vi "Switch Plugin Subpanel.vi"(8 "error in (no error)":errorcluster, 9 "Calling VI":refnum<vi>, 10 "Plugin Info":T1 {"Node Status"."Monitor Doubles"."4" format="%#_9g"; "Node Status"."Monitor Doubles"."3" format="%#_9g"; "Node Status"."Monitor Doubles"."2" format="%#_9g"; "Node Status"."Monitor Doubles"."1" format="%#_9g"; "Node Status"."Timing Statistics (us)"."Period"."Avg" format="%_6g"}, 11 "CIF_UI in":refnum<class "CIF_Manager_UI.lvclass">) -> (0 "error out":errorcluster, 1 "Remove Subpanel":bool, 2 "VI Reference":refnum<vi>, 3 "CIF_UI out":refnum<class "CIF_Manager_UI.lvclass">)   [LabVIEW 2021, in "CIF_Manager_UI.lvclass"]
uses:
  CIF_Manager_UI.lvclass
  C:/Program Files/National Instruments/LabVIEW 2021/vi.lib/CIF Foundation/CIF Core/CIFUI/CIF_UI.lvclass
  Typedef/PluginInfo.ctl
  <vilib>/CIF Foundation/CIF Core/CIFCore/Common/Typedef/Version Simple.ctl
  <vilib>/CIF Foundation/CIF Core/CIFCore/Common/Typedef/gRPC Reported Plugin Status.ctl
  <vilib>/CIF Foundation/CIF Core/CIFCore/Common/Typedef/Plugin State.ctl
  <vilib>/CIF Foundation/CIF Core/CIFCore/Common/Typedef/Timing Statistics.ctl
  <vilib>/CIF Foundation/CIF Core/CIFCore/Common/Typedef/Timing Stats Base.ctl
  <vilib>/CIF Foundation/CIF Core/CIFCore/Common/Typedef/FIFO Statistics.ctl
  <vilib>/CIF Foundation/CIF Core/CIFCore/Common/Typedef/Simple Error.ctl
  <vilib>/CIF Foundation/CIF Core/CIFCore/Common/Typedef/Monitor Doubles.ctl
  <vilib>/CIF Foundation/CIF Core/CIFCore/Common/Typedef/Monitor U64.ctl
  <vilib>/CIF Foundation/CIF Core/CIFCore/Common/Typedef/Monitor I64.ctl
  <vilib>/CIF Foundation/CIF Core/CIFUI/CIF_UI.lvclass/CIF_UI.ctl
  <vilib>/CIF Foundation/CIF Core/CIFUI/Accessors/Read Plugin Subpanel Map.vi
  <vilib>/Utility/LVLibp/Get Exported File List.vi
  <vilib>/Utility/LVLibp/Get Exported File Path.vi
  <vilib>/Utility/LVLibp/Packed Library Path.vi
  <vilib>/CIF Foundation/CIF Core/CIFUI/CIF_UI.lvclass
  <vilib>/CIF Foundation/CIF Core/CIFCore/Common/CIFCoreCommon.lvlib
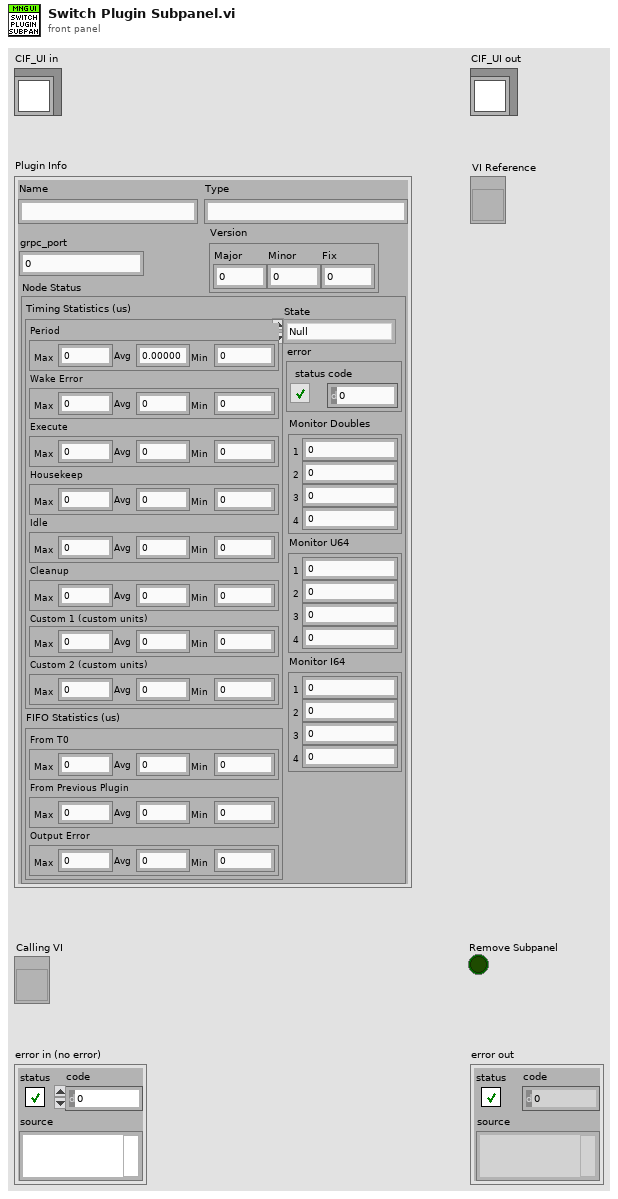
[diagram p1: front panel]
types:
  T1 = typedef "CIF_Manager_UI.lvclass/PluginInfo.ctl" = cluster{"Name":string, "Type":string, "grpc_port":i32, "Version":T2, "Node Status":T3}
  T2 = typedef "CIFCoreCommon.lvlib/Version Simple.ctl" = cluster{"Major":i32, "Minor":i32, "Fix":i32}
  T3 = typedef "CIFCoreCommon.lvlib/gRPC Reported Plugin Status.ctl" = cluster{"State":T4, "Timing Statistics (us)":T5, "FIFO Statistics (us)":T7, "error":T8, "Monitor Doubles":T9, "Monitor U64":T10, "Monitor I64":T11}
  T4 = typedef "CIFCoreCommon.lvlib/Plugin State.ctl" = enum32{"Null", "Creating", "Listening", "Running", "CleaningUp", "Destroying", "Prepared", "FTE_Run"}
  T5 = typedef "CIFCoreCommon.lvlib/Timing Statistics.ctl" = cluster{"Period":T6, "Wake Error":T6, "Execute":T6, "Housekeep":T6, "Idle":T6, "Cleanup":T6, "Custom 1 (custom units)":T6, "Custom 2 (custom units)":T6}
  T6 = typedef "CIFCoreCommon.lvlib/Timing Stats Base.ctl" = cluster{"Max":i64, "Avg":dbl, "Min":i64}
  T7 = typedef "CIFCoreCommon.lvlib/FIFO Statistics.ctl" = cluster{"From T0":T6, "From Previous Plugin":T6, "Output Error":T6}
  T8 = typedef "CIFCoreCommon.lvlib/Simple Error.ctl" = cluster{"status":bool, "code":i32}
  T9 = typedef "CIFCoreCommon.lvlib/Monitor Doubles.ctl" = cluster{"1":dbl, "2":dbl, "3":dbl, "4":dbl}
  T10 = typedef "CIFCoreCommon.lvlib/Monitor U64.ctl" = cluster{"1":u64, "2":u64, "3":u64, "4":u64}
  T11 = typedef "CIFCoreCommon.lvlib/Monitor I64.ctl" = cluster{"1":i64, "2":i64, "3":i64, "4":i64}
  T12 = typedef "CIF_UI.lvclass/Plugin Subpanel Map.ctl" = map{i32, T13}
  T13 = typedef "CIF_UI.lvclass/Subpanel Data.ctl" = cluster{"VI Reference":refnum<vi>, "Plugin Subpanel Events":T14}
  T14 = typedef "CIF_UI.lvclass/Plugin Subpanel Events.ctl" = cluster{"Plugin Shutdown":refnum<user-event>}
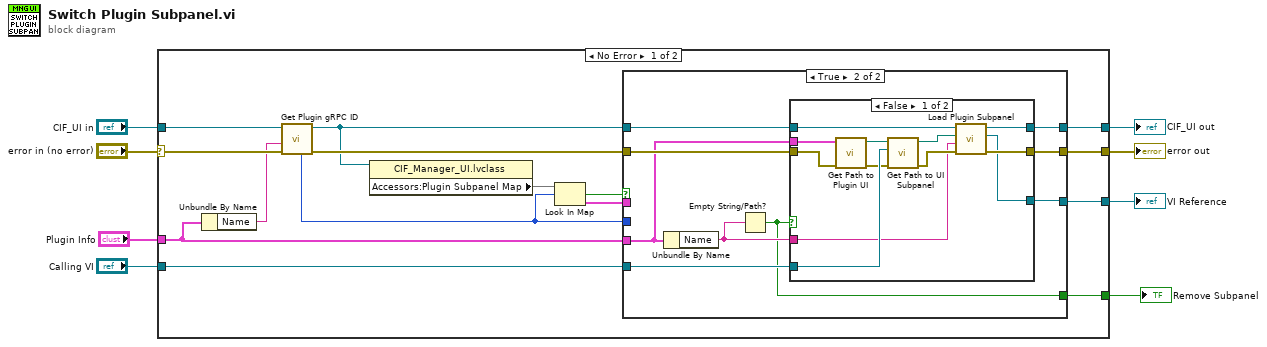
[diagram p0: block diagram]
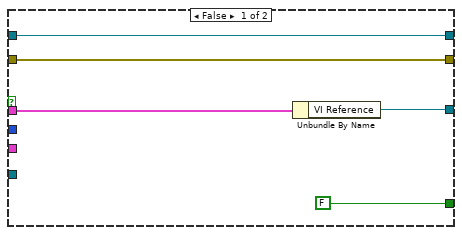
[diagram p2: hidden frame]
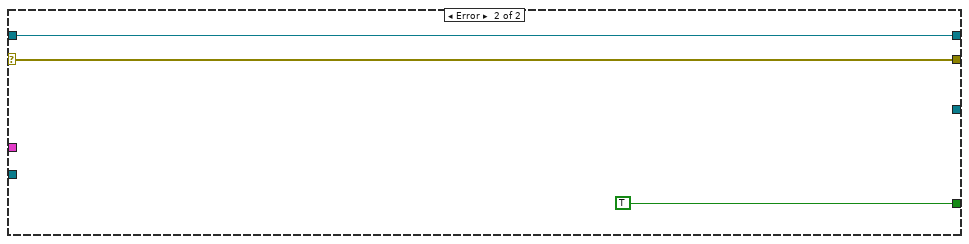
[diagram p4: hidden frame]
diagram:
  n1 = case shown="No Error" "error in (no error)" {
    selector: "error in (no error)" -> [w17 w54]
    tunnel: [w20 w54] -> w7
    tunnel: [w21 w53] -> w5
    tunnel: "CIF_UI in" -> [w18 w53]
    tunnel: [w19 _] -> w4
    tunnel: "Plugin Info" -> [w12 _]
    tunnel: "Calling VI" -> [w13 _]
    tunnel: [w11 TRUE] -> w1
    frame No Error {
      n2 = Unbundle By Name(w12) -> ("Name"=w14:string)
      n3 = call <vilib>:"Get Plugin gRPC ID.vi"("error in (no error)"=w17, "Plugin Name"=w14, "CIF_UI in"=w18) -> ("error out"=w16:errorcluster, "CIF_UI out"=w10:refnum<class "CIF_Manager_UI.lvclass">, "gRPC Port"=w15:i32)  [unwired: 4 in, 2 out]
      n4 = property class="CIF_Manager_UI.lvclass"(reference=w10) -> ("Accessors:Plugin Subpanel Map"=w9:T12)  [unwired: 1 in, 2 out]
      n5 = Look In Map(map=w9, key=w15) -> (key not found?=w23:bool, value=w22:T13)  [unwired: 1 in]
      n6 = case shown="True" w23 {
        tunnel: w22 -> [w28 _]
        tunnel: w10 -> [w27 w37]
        tunnel: w15 -> [_ _]
        tunnel: [w27 w34] -> w21
        tunnel: w16 -> [w26 w32]
        tunnel: [w26 w36] -> w20
        tunnel: [w25 w35] -> w19
        tunnel: w13 -> [_ w33]
        tunnel: w12 -> [_ w31]
        tunnel: [FALSE w29] -> w11
        frame False {
          n7 = Unbundle By Name(w28) -> ("VI Reference"=w25:refnum<vi>)
        }
        frame True {
          n8 = Unbundle By Name(w31) -> ("Name"=w30:string)
          n9 = Empty String/Path?(string/path=w30) -> (empty?=w29:bool)
          n10 = case shown="False" w29 {
            tunnel: w37 -> [w49 w51]
            tunnel: [w48 w50] -> w36
            tunnel: [w47 _] -> w35
            tunnel: [w46 w51] -> w34
            tunnel: w33 -> [w45 _]
            tunnel: w32 -> [w44 w50]
            tunnel: w31 -> [w40 _]
            tunnel: w30 -> [w39 _]
            frame False {
              n11 = call "Get Path to Plugin UI.vi"("error in (no error)"=w44, "Plugin Info"=w40) -> ("error out"=w38:errorcluster, "Plugin UI Path"=w42:path)  [unwired: 8 in]
              n12 = call "Get Path to UI Subpanel.vi"("error in (no error)"=w38, "Calling VI"=w45, "packed library path"=w42) -> ("error out"=w43:errorcluster, "Path to Subpanel"=w41:path)  [unwired: 7 in]
              n13 = call <vilib>:"Load Plugin Subpanel.vi"("error in (no error)"=w43, "Plugin Name"=w39, "Path"=w41, "CIF_UI in"=w49) -> ("error out"=w48:errorcluster, "VI Reference"=w47:refnum<vi>, "CIF_UI out"=w46:refnum<class "CIF_Manager_UI.lvclass">)  [unwired: 5 in]
            }
            frame True {
            }
          }
        }
      }
    }
    frame Error {
    }
  }
  "error out" <- w7
  "CIF_UI out" <- w5
  "VI Reference" <- w4
  "Remove Subpanel" <- w1
